vi "Test COMport Name.vi"() -> ()   [LabVIEW 2018, in "Application.lvlib"]
uses:
  Application.lvlib
  <vilib>/Instr/_visa.llb/VISA Configure Serial Port (Instr).vi
panel:
  in  "Stop Button":bool
  in  "VISA resource name":refnum<visa-resource-name>
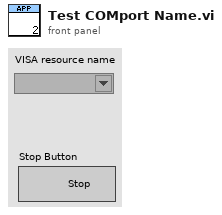
[diagram p1: front panel]
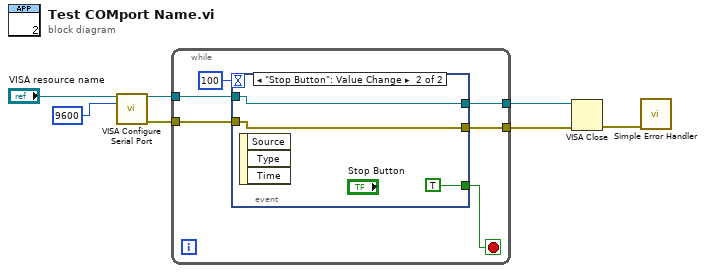
[diagram p0: block diagram]
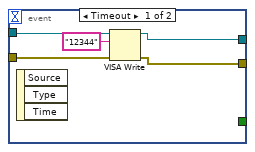
[diagram p2: hidden frame]
diagram:
  n1 = call-poly "VISA Configure Serial Port"("VISA resource name"="VISA resource name", "baud rate (9600)"=u32 9600) -> ("VISA resource name out"=w5:refnum<visa-resource-name>, "error out"=w4:errorcluster)  [unwired: 12 in]
  n2 = while {
    tunnel: w5 -> [w12]
    tunnel: w4 -> [w11]
    tunnel: [w10] -> w3
    tunnel: [w9] -> w2
    stop <- w8 stop-if-true
    n3 = event shown="[1] \"Stop Button\": Value Change" {
      selector: _ -> [_ _]
      dyn-events: _ -> [_ _]
      timeout: 100 -> [_ _]
      tunnel: w12 -> [w18 w20]
      tunnel: w11 -> [w17 w19]
      tunnel: [w16 w19] -> w10
      tunnel: [w15 w20] -> w9
      tunnel: [_ TRUE] -> w8
      event Timeout {
        n4 = event-data() -> ()  [unwired: 1 in, 3 out]
        n5 = VISA Write(VISA resource name=w18, write buffer="12344", error in (no error)=w17) -> (VISA resource name out=w15:refnum<visa-resource-name>, error out=w16:errorcluster)  [unwired: 1 out]
      }
      event "Stop Button": Value Change {
        n6 = event-data() -> ()  [unwired: 1 in, 3 out]
      }
    }
  }
  n7 = VISA Close(VISA resource name=w2, error in (no error)=w3) -> (error out=w1:errorcluster)
  n8 = call <vilib>:"Simple Error Handler.vi"("error in (no error)"=w1) -> ()  [unwired: 4 in, 5 out]
